vi "p8.6.vi"() -> ()   [LabVIEW 2020]
uses:
  <vilib>/vision/NI_Vision_Development_Module.lvlib
panel:
  out "FFT Imagen1":T1(plugin-control)
  in  "FFT Image Type":T2=3 items=["Grayscale (U8)", "Grayscale (I16)", "Grayscale (SGL)", "Complex (CSG)", "RGB (U32)", "HSL (U32)", "RGB (U64)", "Grayscale (U16)"]
  out "Imagen1":T1(plugin-control)
  in  "Image Type":T2 items=["Grayscale (U8)", "Grayscale (I16)", "Grayscale (SGL)", "Complex (CSG)", "RGB (U32)", "HSL (U32)", "RGB (U64)", "Grayscale (U16)"]
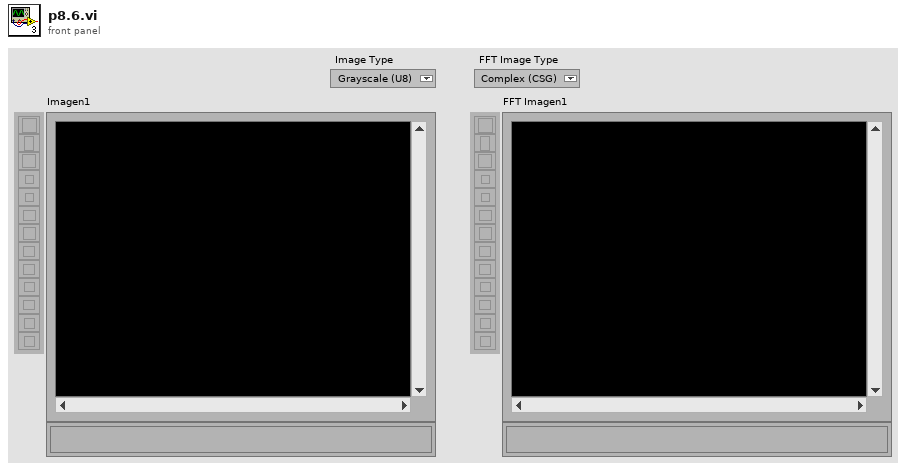
[diagram p1: front panel]
types:
  T1 = typedef "IMAQ Image.ctl" = refnum<image>
  T2 = typedef "Image Type" = u32
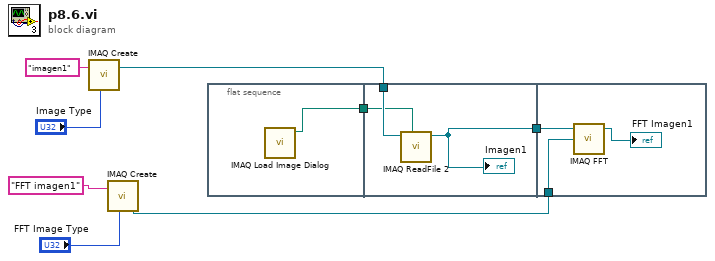
[diagram p0: block diagram]
diagram:
  n1 = call "IMAQ Create"("Image Name"="imagen1", "Image Type"="Image Type") -> ("New Image"=w6:T1)  [unwired: 3 in, 1 out]
  n2 = call "IMAQ Create"("Image Name"="FFT imagen1", "Image Type"="FFT Image Type") -> ("New Image"=w3:T1)  [unwired: 3 in, 1 out]
  n3 = flat-sequence {
    tunnel: [w9] -> w1
    tunnel: w6 -> [w12]
    tunnel: [w11] -> w2
    tunnel: w1 -> [w10]
    tunnel: w3 -> [w15]
    tunnel: w2 -> [w14]
    frame #0 {
      n4 = call "IMAQ Load Image Dialog"() -> ("Path"=w9:path)  [unwired: 9 in, 2 out]
    }
    frame #1 {
      n5 = call "IMAQ ReadFile 2"("File Path"=w10, "Image"=w12) -> ("Image Out"=w11:T1)  [unwired: 5 in, 4 out]
      "Imagen1" <- w11
    }
    frame #2 {
      n6 = call "IMAQ FFT"("Image Dst"=w15, "Image Src"=w14) -> ("Image Dst Out"=→"FFT Imagen1":T1)  [unwired: 2 in, 1 out]
    }
  }
